vi "Apply Steering Frame Velocity to Motors.vi"(6 "constraint error tolerance (1E-12)":dbl=1e-12, 7 "wheel indexes":i32[](array[numeric]), 8 "error in (no error)":errorcluster, 10 "steering frame velocity":dbl[](array[numeric])=[0.0, 0.0, 0.0], 11 "steering frame in":refnum<class "NI_Robotics_Steering Frame.lvclass">) -> (0 "error out":errorcluster, 1 "ccw motor angle setpoints (rad)":dbl[](array[numeric]), 2 "ccw motor velocity setpoints":dbl[](array[numeric]), 3 "steering frame out":refnum<class "NI_Robotics_Steering Frame.lvclass">, 4 "ccw caster motor velocity setpoints":dbl[](array[numeric]))   [LabVIEW 2017, in "NI_Robotics_Steering Frame.lvclass"]
doc: "Calculates the velocity and angle of each motor necessary to satisfy the <B>steering frame velocity</B> or <B>arc velocity</B> at the center of a steering frame. You must manually select the polymorphic instance to use."
uses:
  <vilib>/robotics/Steering/Steering Frame/NI_Robotics_Steering Frame.lvclass
  <vilib>/robotics/Steering/Steering Frame/NI_Robotics_Steering Frame.lvclass/NI_Robotics_Steering Frame.ctl
  <vilib>/robotics/Steering/Wheel/NI_Robotics_Wheel.lvclass/NI_Robotics_Wheel.ctl
  <vilib>/robotics/Utilities/Generate Error.vi
  <vilib>/robotics/Steering/Wheel/Convert Steering Frame Velocity to Wheel Frame.vi
  <vilib>/robotics/Steering/Wheel/Apply Wheel State to Motors.vi
  <vilib>/robotics/Steering/Wheel/Create Wheel Angular Velocity Row_Frame.vi
  <vilib>/robotics/Steering/Wheel/Create Caster Angular Velocity Row_Frame.vi
  <vilib>/robotics/Steering/Wheel/Get Motor Velocity Setpoint_Frame.vi
  <vilib>/robotics/Steering/Wheel/Get Steering Motor Angle Setpoint_Frame.vi
  <vilib>/robotics/Steering/Wheel/Get Caster Motor Velocity Setpoint_Frame.vi
  <vilib>/Analysis/baseanly.llb/A x Vector.vi
  <vilib>/robotics/Steering/Wheel/Get Motor Velocity Setpoint.vi
  <vilib>/robotics/Steering/Wheel/NI_Robotics_Wheel.lvclass
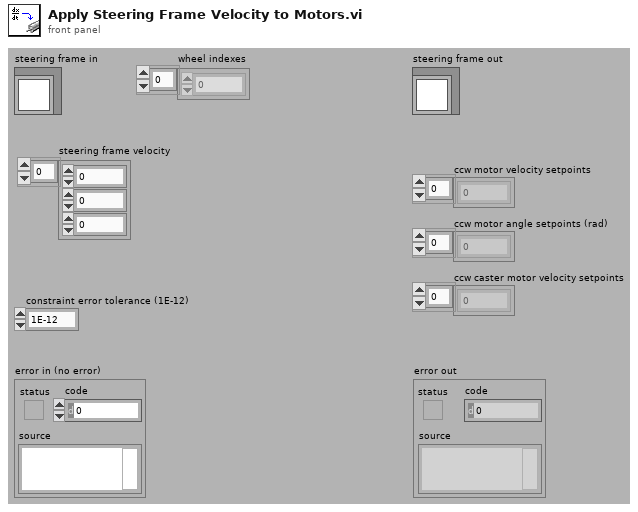
[diagram p1: front panel]
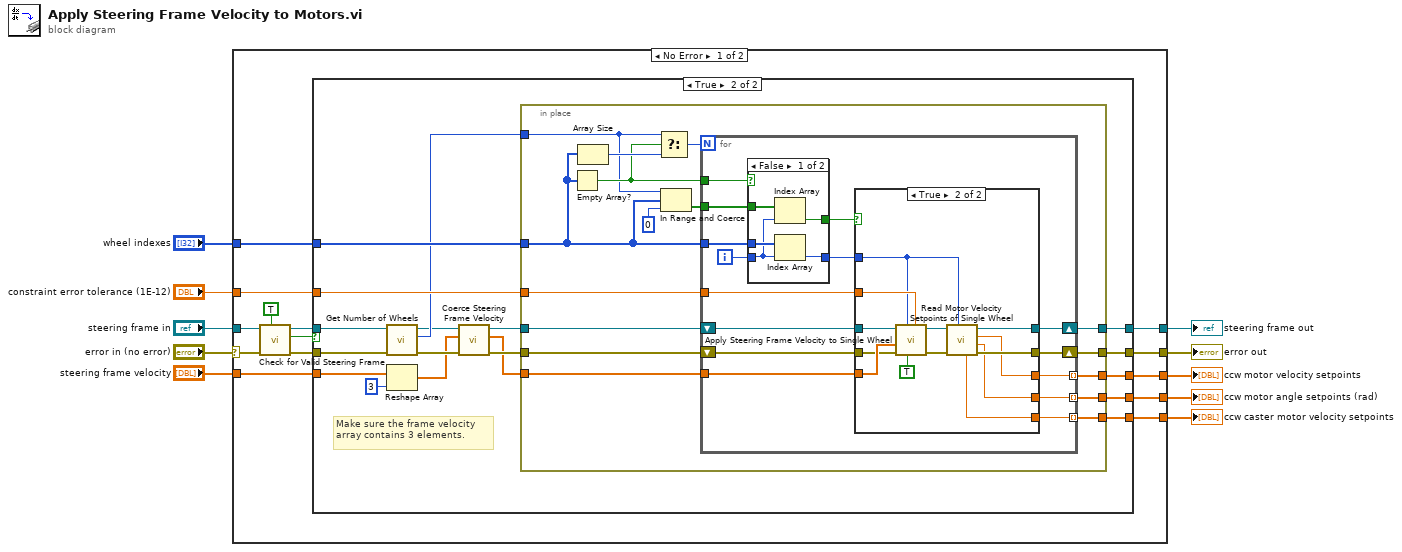
[diagram p0: block diagram]
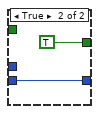
[diagram p4: hidden frame]
diagram:
  n1 = case shown="No Error" "error in (no error)" {
    selector: "error in (no error)" -> [w18 w99]
    tunnel: [w23 w99] -> w4
    tunnel: [w22 w98] -> w5
    tunnel: "steering frame in" -> [w20 w98]
    tunnel: "steering frame velocity" -> [w21 _]
    tunnel: "constraint error tolerance (1E-12)" -> [w24 _]
    tunnel: "wheel indexes" -> [w14 _]
    tunnel: [w13 _] -> w3
    tunnel: [w12 _] -> w2
    tunnel: [w11 _] -> w1
    frame No Error {
      n2 = call <vilib>:"Check for Valid Steering Frame.vi"("produce error if invalid (T)"=TRUE, "error in (no error)"=w18, "steering frame in"=w20) -> ("error out"=w17:errorcluster, "valid?"=w16:bool, "steering frame out"=w19:refnum<class "NI_Robotics_Steering Frame.lvclass">)  [unwired: 6 in]
      n3 = case shown="True" w16 {
        tunnel: w24 -> [_ w44]
        tunnel: [w25 w37] -> w23
        tunnel: [w26 w38] -> w22
        tunnel: w21 -> [_ w41]
        tunnel: w19 -> [w26 w35]
        tunnel: w17 -> [w25 w33]
        tunnel: w14 -> [_ w40]
        tunnel: [_ w30] -> w13
        tunnel: [_ w29] -> w12
        tunnel: [_ w28] -> w11
        frame False {
        }
        frame True {
          # "Make sure the frame velocity array contains 3 elements."
          n4 = call <vilib>:"Get Number of Wheels.vi"("error in (no error)"=w33, "steering frame in"=w35) -> ("error out"=w32:errorcluster, "number of wheels"=w36:i32, "steering frame out"=w34:refnum<class "NI_Robotics_Steering Frame.lvclass">)  [unwired: 7 in]
          n5 = Reshape Array(w41, 3 ("dimension size")) -> (w31:dbl[])
          n6 = call-dynamic "Coerce Steering Frame Velocity.vi"("error in (no error)"=w32, "steering frame velocity"=w31, "steering frame in"=w34) -> ("error out"=w43:errorcluster, "coerced steering frame velocity"=w27:dbl[], "steering frame out"=w39:refnum<class "NI_Robotics_Steering Frame.lvclass">)  [unwired: 6 in]
          n7 = in-place {
            in-place-border: w44 -> [w60]
            in-place-border: w43 -> [w59]
            in-place-border: [w58] -> w37
            in-place-border: w27 -> [w57]
            in-place-border: w40 -> [w53]
            in-place-border: w36 -> [w50]
            in-place-border: w39 -> [w49]
            in-place-border: [w48] -> w38
            in-place-border: [w47] -> w30
            in-place-border: [w46] -> w29
            in-place-border: [w45] -> w28
            n8 = Empty Array?(array=w53) -> (empty?=w54:bool)
            n9 = Array Size(array=w53) -> (size(s)=w55:i32)
            n10 = Select(t=w50, s=w54, f=w55) -> (s? t:f=w56:i32)
            n11 = In Range and Coerce(upper limit=w50, x=w53, lower limit=0) -> (In Range?=w51:bool[])  [unwired: 1 out]
            n12 = for {
              N: w56 -> [_]
              tunnel: w60 -> [w75]
              tunnel: w57 -> [w74]
              shift-right: [w72] -> w58
              shift-left: w59 -> [w73]
              tunnel: w53 -> [w70]
              tunnel: w54 -> [w71]
              tunnel: w51 -> [w67]
              shift-right: [w64] -> w48
              shift-left: w49 -> [w65]
              tunnel: [w63] -> w47 mode=indexing
              tunnel: [w62] -> w46 mode=indexing
              tunnel: [w61] -> w45 mode=indexing
              i -> [w69]
              n13 = case shown="False" w71 {
                tunnel: w70 -> [w95 _]
                tunnel: w69 -> [w93 w97]
                tunnel: [w92 w97] -> w68
                tunnel: w67 -> [w94 _]
                tunnel: [w91 TRUE ("lower limit")] -> w66
                frame False {
                  n14 = Index Array(array=w94, index=w93) -> (element=w91:bool)
                  n15 = Index Array(array=w95, index=w93) -> (element=w92:i32)
                }
                frame True {
                }
              }
              n16 = case shown="True" w66 {
                tunnel: w75 -> [_ w89]
                tunnel: w74 -> [_ w90]
                tunnel: w73 -> [w77 w88]
                tunnel: [w77 w81] -> w72
                tunnel: w68 -> [_ w83]
                tunnel: w65 -> [w76 w87]
                tunnel: [w76 w84] -> w64
                tunnel: [_ w80] -> w63
                tunnel: [_ w79] -> w62
                tunnel: [_ w78] -> w61
                frame False {
                }
                frame True {
                  n17 = call <vilib>:"Apply Steering Frame Velocity to Single Wheel.vi"("constraint error tolerance (1E-12)"=w89, "apply data to motors"=TRUE, "wheel index"=w83, "error in (no error)"=w88, "steering frame velocity"=w90, "steering frame in"=w87) -> ("error out"=w82:errorcluster, "steering frame out"=w85:refnum<class "NI_Robotics_Steering Frame.lvclass">)  [unwired: 4 in]
                  n18 = call <vilib>:"Read Motor Velocity Setpoints of Single Wheel.vi"("wheel index"=w83, "error in (no error)"=w82, "steering frame in"=w85) -> ("error out"=w81:errorcluster, "ccw motor angle setpoint (rad)"=w79:dbl, "ccw motor velocity setpoint"=w80:dbl, "steering frame out"=w84:refnum<class "NI_Robotics_Steering Frame.lvclass">, "ccw caster motor velocity setpoint"=w78:dbl)  [unwired: 4 in]
                }
              }
            }
          }
        }
      }
    }
    frame Error {
    }
  }
  "error out" <- w4
  "steering frame out" <- w5
  "ccw motor velocity setpoints" <- w3
  "ccw motor angle setpoints (rad)" <- w2
  "ccw caster motor velocity setpoints" <- w1
